vi "Main.vi"() -> ()   [LabVIEW 2019]
uses:
  <vilib>/vision/Image Controls.llb/IMAQ Image.ctl
  <vilib>/vision/NI_Vision_Development_Module.lvlib
panel:
  in  "Save Button":bool
  in  "Clear Button":bool
  in  "Image Path":path=path "Data/(1).jpg" caption="Picture Path"
  in  "Exit":bool
  in  "Start":bool
  out "Results":string
  out "Image":T1(plugin-control)
  # "Application Panel"
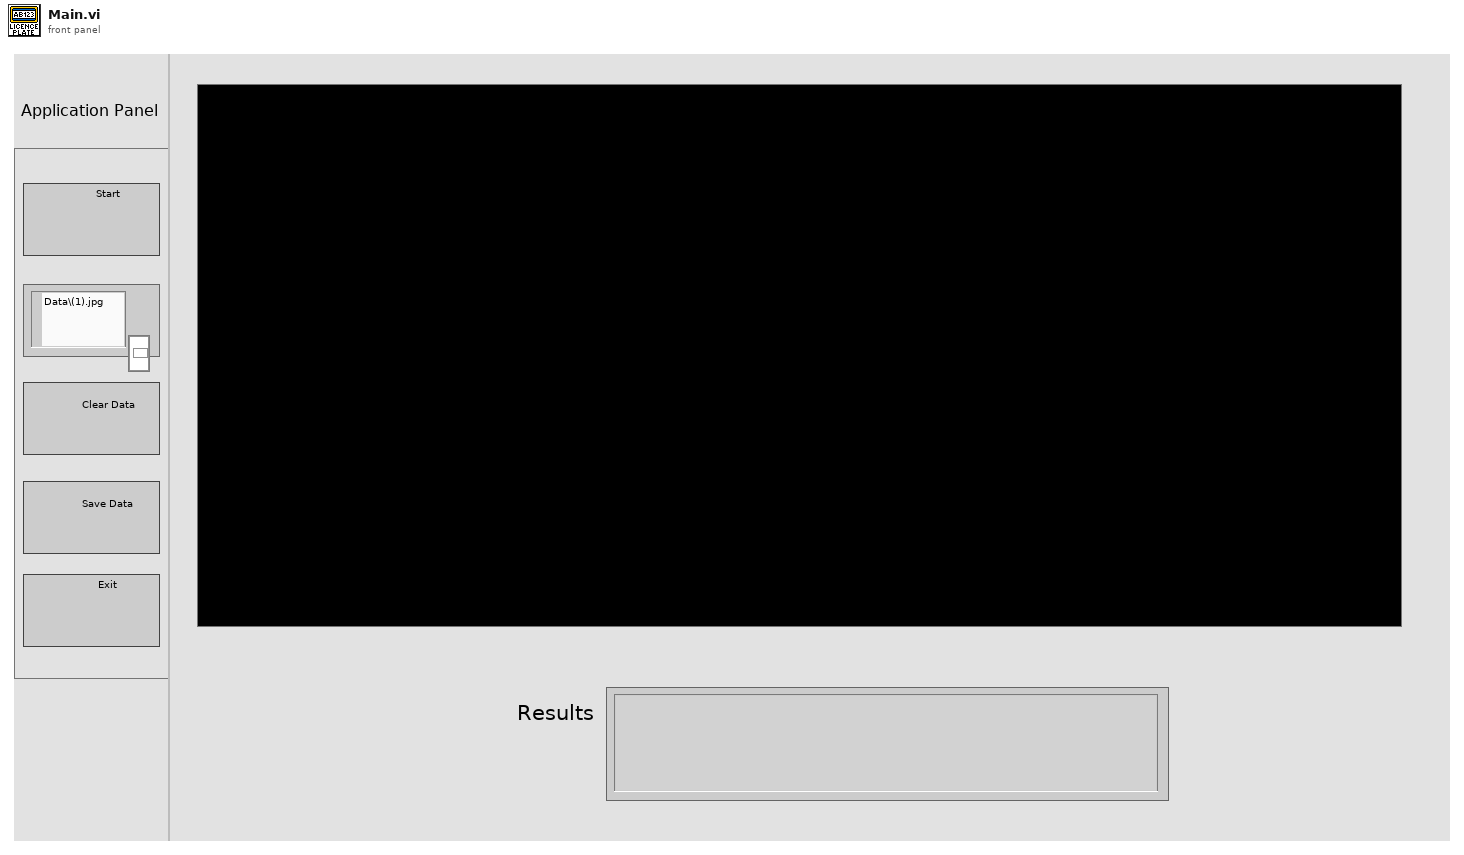
[diagram p1: front panel]
types:
  T1 = typedef "IMAQ Image.ctl" = refnum<image>
  T2 = enum32{"Invalid", "Standard", "Closed", "Hidden", "Minimized", "Maximized"}
  T3 = enum32{"invalid app kind", "Development System", "Run Time System", "Student Edition", "Embedded LabVIEW", "Evaluation", "Custom"}
  T4 = cluster{"Core":cluster{"Current VI Reference":refnum<vi>, "Close Panel on Exit?":bool}, "Your Boolean data":bool, "Results":string, "Image Path":path, "Data":cluster{"Rectangle":i32[]}, "Image":refnum<image>, "Python Path":path}
  T5 = cluster{"Current VI Reference":refnum<vi>, "Close Panel on Exit?":bool}
  T6 = typedef "Image Type" = u32
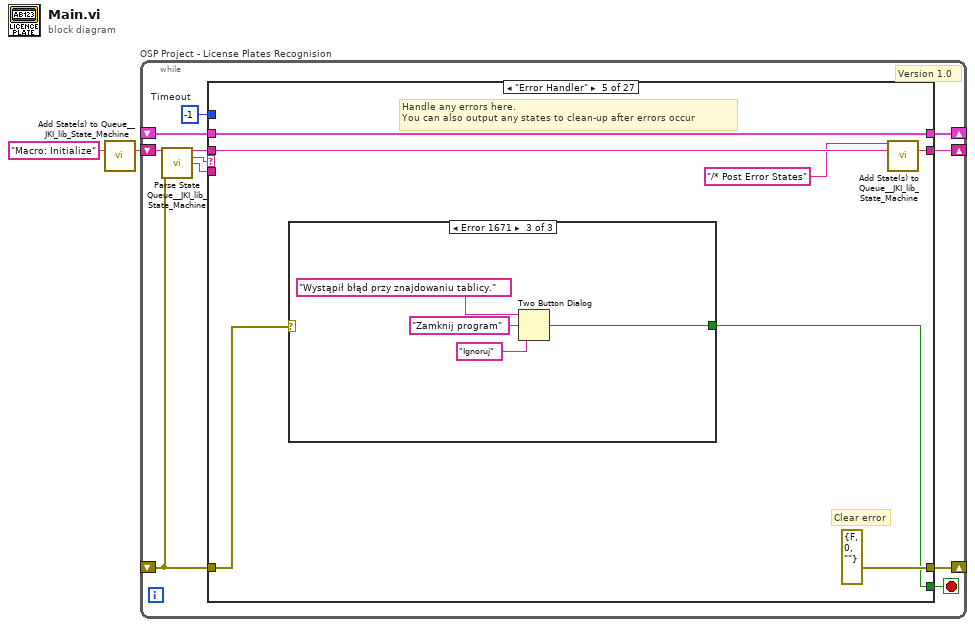
[diagram p0: block diagram]
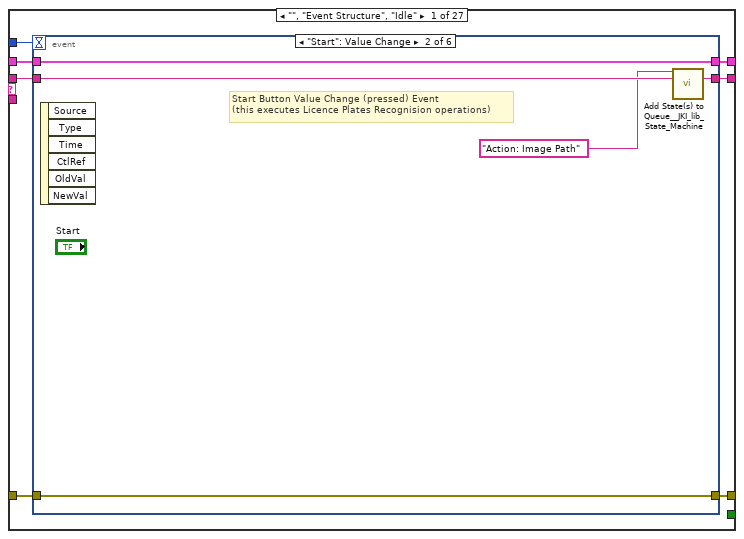
[diagram p2: hidden frame]
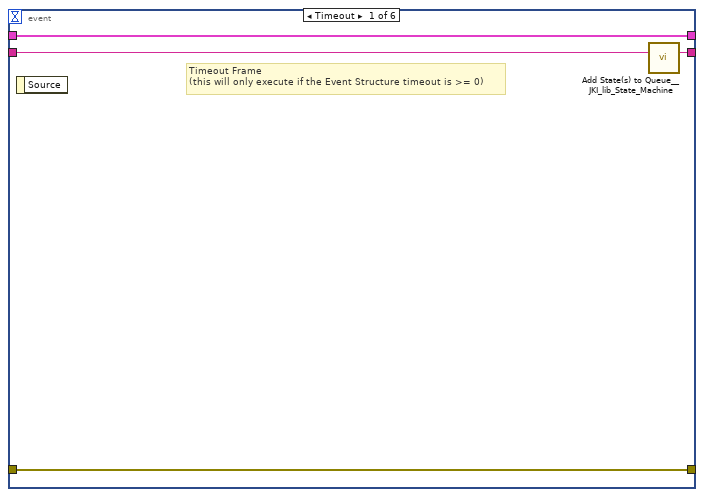
[diagram p3: hidden frame]
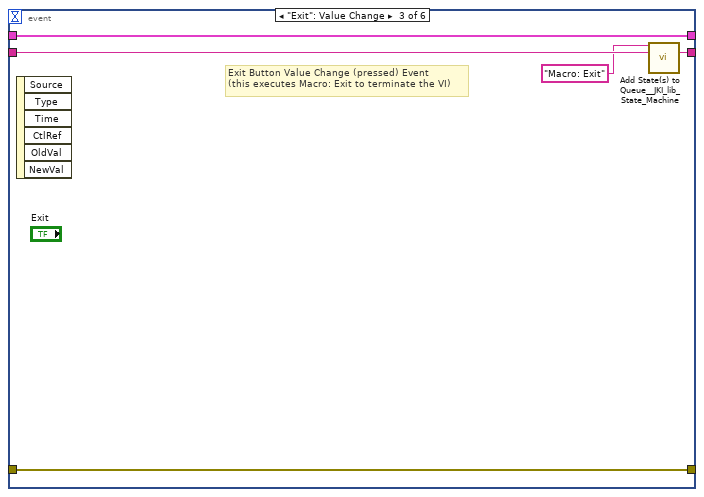
[diagram p4: hidden frame]
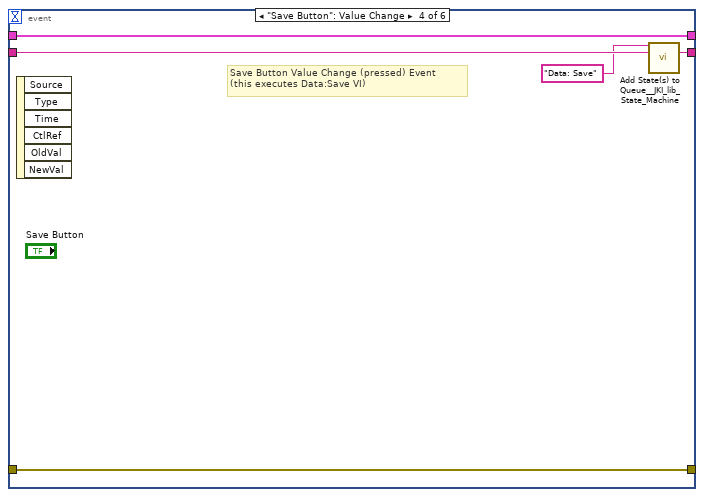
[diagram p5: hidden frame]
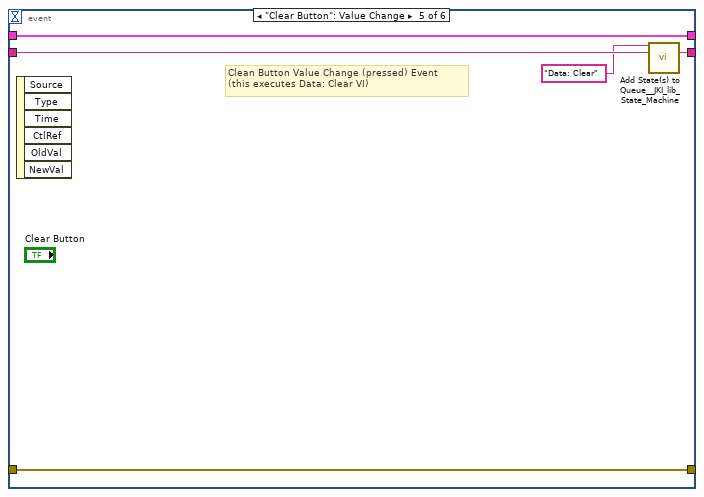
[diagram p6: hidden frame]
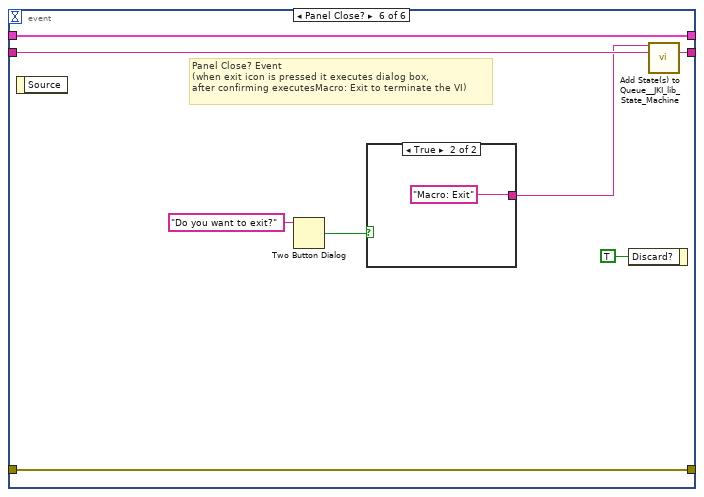
[diagram p7: hidden frame]
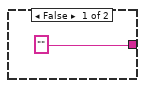
[diagram p8: hidden frame]
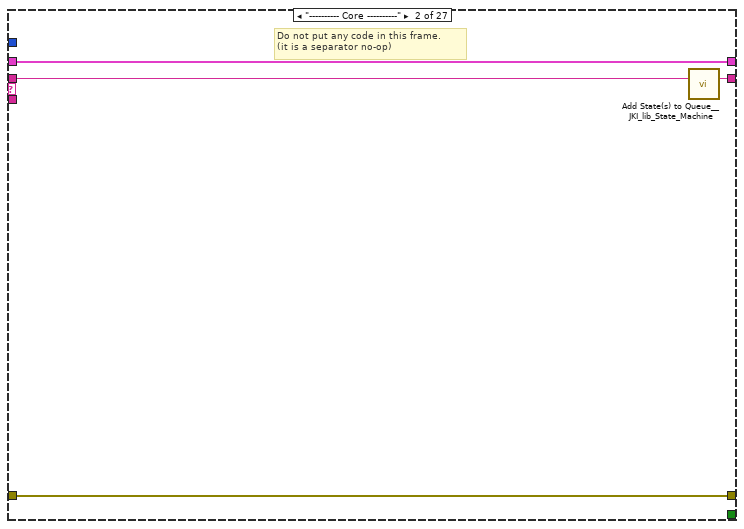
[diagram p9: hidden frame]
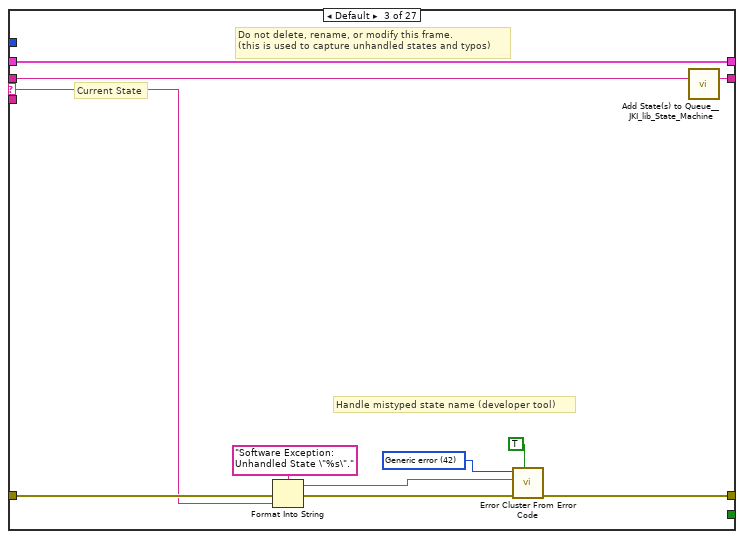
[diagram p10: hidden frame]
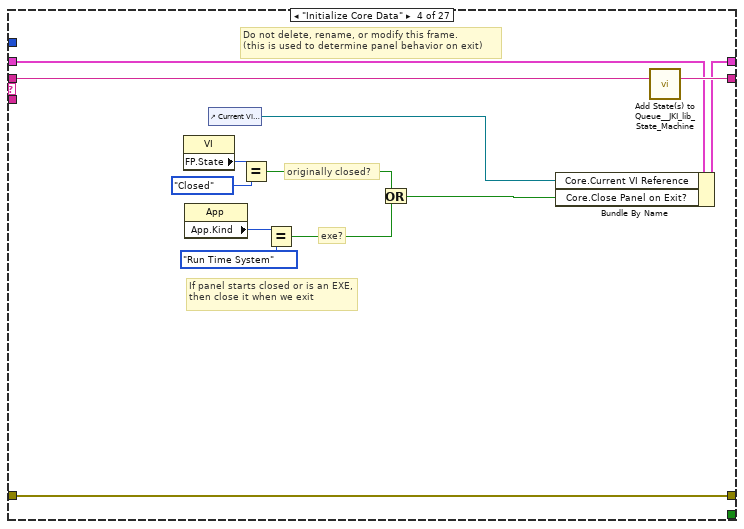
[diagram p11: hidden frame]
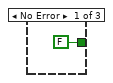
[diagram p12: hidden frame]
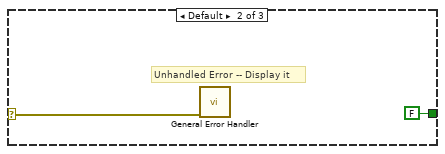
[diagram p13: hidden frame]
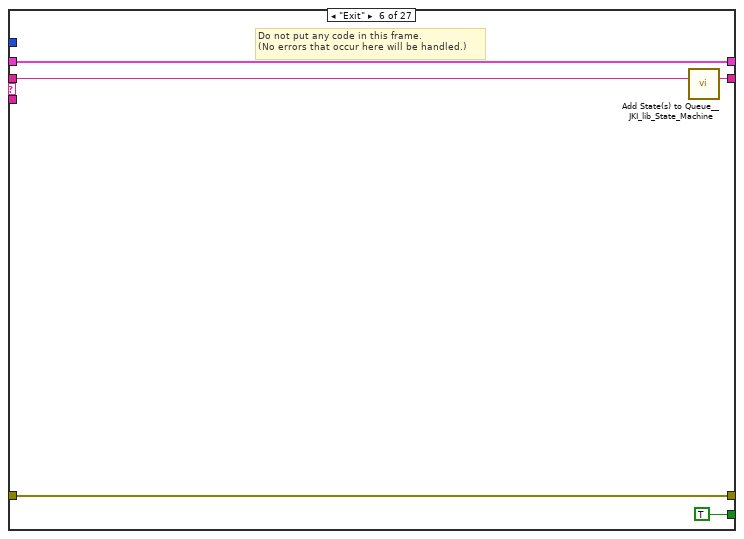
[diagram p14: hidden frame]
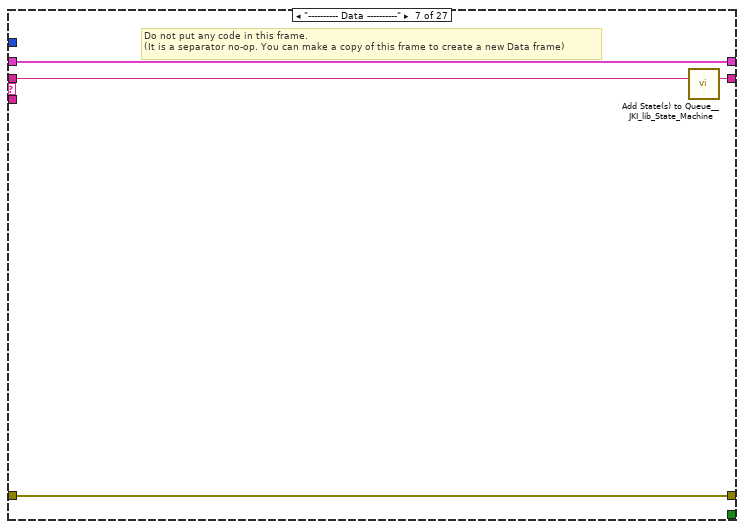
[diagram p15: hidden frame]
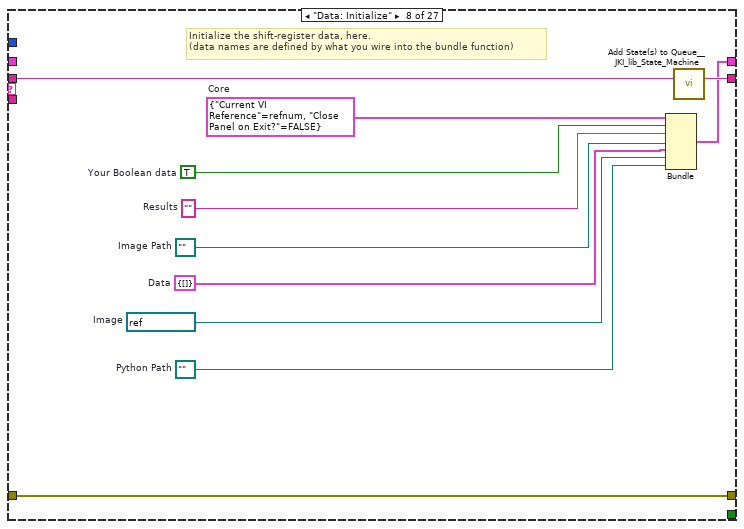
[diagram p16: hidden frame]
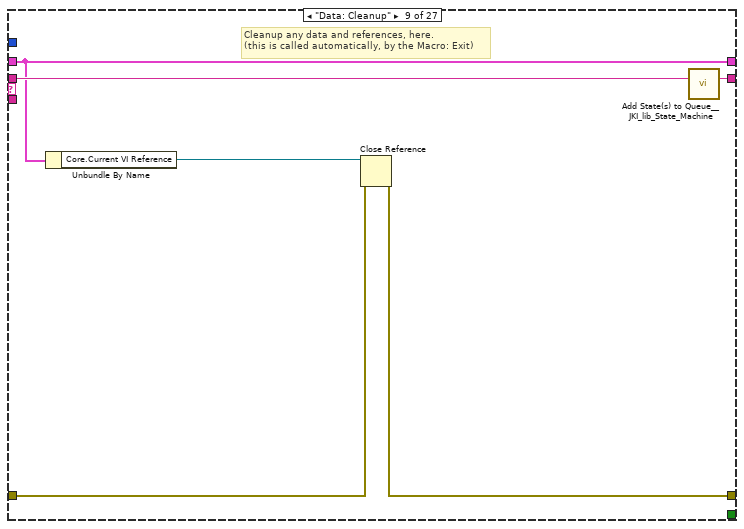
[diagram p17: hidden frame]
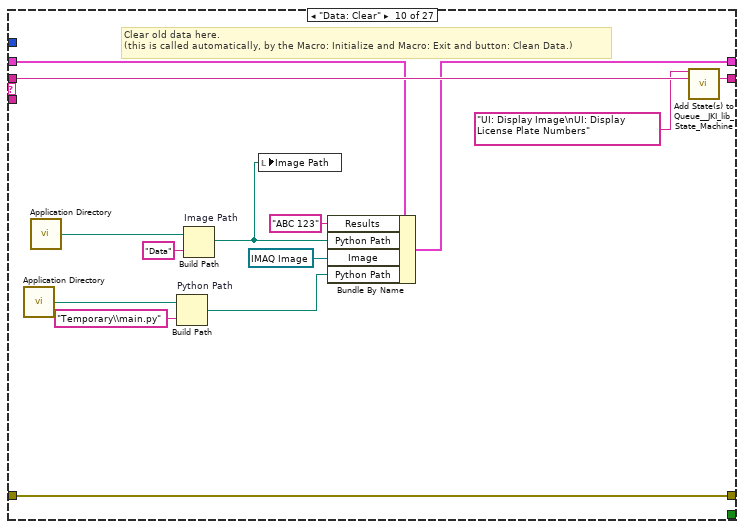
[diagram p18: hidden frame]
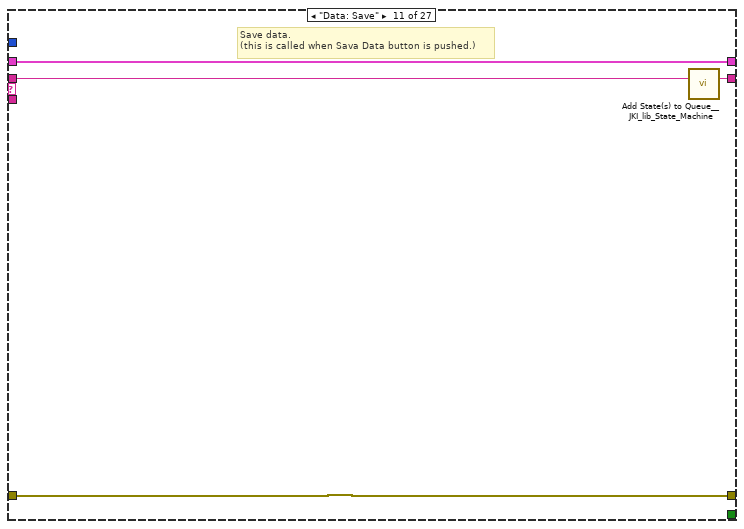
[diagram p19: hidden frame]
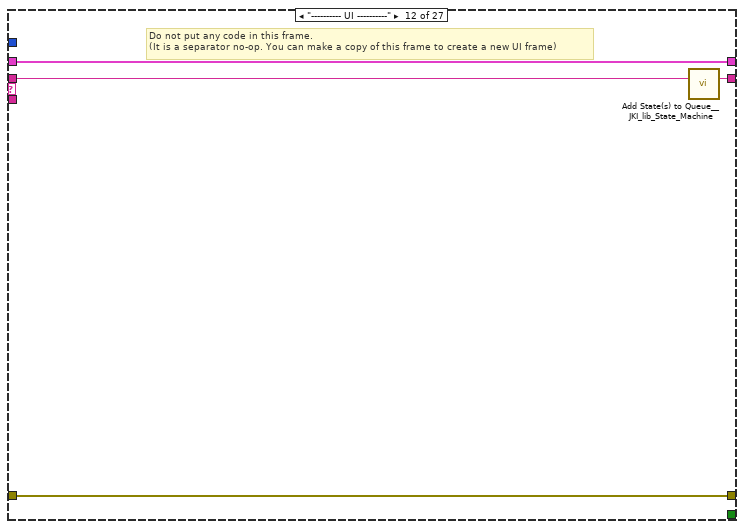
[diagram p20: hidden frame]
diagram:
  n1 = call <vilib>:"Add State(s) to Queue__JKI_lib_State_Machine.vi"("State(s) in (\"\")"="Macro: Initialize") -> ("States Out"=w2:string)  [unwired: 14 in]
  n2 = while "OSP Project - License Plates Recognision" {
    shift-right: [w6] -> _
    shift-left: _ -> [w5]
    shift-right: [w9] -> _
    shift-left: _ -> [w3]
    shift-right: [w8] -> _
    shift-left: w2 -> [w10]
    stop <- w7 stop-if-true
    w4 = -1  # Timeout
    # "Version 1.0"
    n3 = call <vilib>:"Parse State Queue__JKI_lib_State_Machine.vi"("State Queue"=w10, "Error In (no error)"=w3) -> ("Remaining States"=w12:string, "Current State"=w13:string, "Arguments"=w11:string)  [unwired: 11 in]
    n4 = case shown="\"Error Handler\"" w13 {
      selector: w13 -> [_ _ w59 _ _ _ _ _ _ _ _ _ _ _ _ _ _ _ _ _ _ _ _ _ _ _ _]
      tunnel: w12 -> [w20 w58 w63 w82 w89 w101 w105 w116 w122 w136 w140 w144 w148 w154 w165 w235 w240 w244 w249 w259 w263 w273 w300 w309 w318 w329 w338]
      tunnel: w11 -> [_ _ _ _ _ _ _ _ _ _ _ _ _ w149 w159 _ _ _ _ _ _ _ _ _ _ _ _]
      tunnel: w5 -> [w18 w55 w61 w75 w86 w99 w102 _ w117 w132 w138 w141 w146 w152 w161 w232 w237 w241 w246 w256 w260 w269 w288 w303 w313 w321 w332]
      tunnel: [w17 w56 w65 w79 errorcluster {"status"=FALSE, "code"=0, "source"=""} ("error out") w98 w103 w113 w118 w134 w137 w142 w145 w150 w162 w233 w238 w242 w247 w257 w261 w271 w283 w307 w316 w327 w335] -> w9
      tunnel: w3 -> [w16 w56 w64 w79 w84 w98 w103 w113 w119 w134 w137 w142 w145 w151 w163 w233 w238 w242 w247 w257 w261 w271 w286 w307 w316 w327 w334]
      tunnel: [w19 w57 w62 w81 w88 w100 w104 w115 w121 w135 w139 w143 w147 w153 w164 w234 w239 w243 w248 w258 w262 w272 w299 w308 w317 w328 w337] -> w8
      tunnel: [_ _ _ _ w83 TRUE _ _ _ _ _ _ _ _ _ _ _ _ _ _ _ _ _ _ _ _ _] -> w7
      tunnel: [w15 w55 w61 w80 w86 w99 w102 w114 w117 w133 w138 w141 w146 w152 w161 w232 w237 w241 w246 w256 w260 w270 w289 w304 w314 w322 w333] -> w6
      tunnel: w4 -> [w14 _ _ _ _ _ _ _ _ _ _ _ _ _ _ _ _ _ _ _ _ _ _ _ _ _ _]
      frame "", "Event Structure", "Idle" {
        n5 = event shown="[1] \"Start\": Value Change" {
          selector: _ -> [_ _ _ _ _ _]
          dyn-events: _ -> [_ _ _ _ _ _]
          timeout: w14 -> [_ _ _ _ _ _]
          tunnel: w20 -> [w24 w29 w34 w39 w44 w52]
          tunnel: [w23 w28 w33 w38 w43 w51] -> w19
          tunnel: w18 -> [w21 w26 w31 w36 w41 w49]
          tunnel: [w22 w27 w32 w37 w42 w50] -> w17
          tunnel: w16 -> [w22 w27 w32 w37 w42 w50]
          tunnel: [w21 w26 w31 w36 w41 w49] -> w15
          event Timeout {
            # "Timeout Frame\n(this will only execute if the Event Structure timeout is >= 0)"
            n6 = event-data() -> ()  [unwired: 1 in, 1 out]
            n7 = call <vilib>:"Add State(s) to Queue__JKI_lib_State_Machine.vi"("State(s) in (\"\")"=w24) -> ("States Out"=w23:string)  [unwired: 14 in]
          }
          event "Start": Value Change {
            # "Start Button Value Change (pressed) Event\n(this executes Licence Plates Recognision operations)"
            n8 = event-data() -> ()  [unwired: 1 in, 6 out]
            n9 = call <vilib>:"Add State(s) to Queue__JKI_lib_State_Machine.vi"("State(s) in Front (\"\")"="Action: Image Path", "State(s) in (\"\")"=w29) -> ("States Out"=w28:string)  [unwired: 13 in]
          }
          event "Exit": Value Change {
            # "Exit Button Value Change (pressed) Event\n(this executes Macro: Exit to terminate the VI)"
            n10 = event-data() -> ()  [unwired: 1 in, 6 out]
            n11 = call <vilib>:"Add State(s) to Queue__JKI_lib_State_Machine.vi"("State(s) in Front (\"\")"="Macro: Exit", "State(s) in (\"\")"=w34) -> ("States Out"=w33:string)  [unwired: 13 in]
          }
          event "Save Button": Value Change {
            # "Save Button Value Change (pressed) Event\n(this executes Data:Save VI)"
            n12 = event-data() -> ()  [unwired: 1 in, 6 out]
            n13 = call <vilib>:"Add State(s) to Queue__JKI_lib_State_Machine.vi"("State(s) in Front (\"\")"="Data: Save", "State(s) in (\"\")"=w39) -> ("States Out"=w38:string)  [unwired: 13 in]
          }
          event "Clear Button": Value Change {
            # "Clean Button Value Change (pressed) Event\n(this executes Data: Clear VI)"
            n14 = event-data() -> ()  [unwired: 1 in, 6 out]
            n15 = call <vilib>:"Add State(s) to Queue__JKI_lib_State_Machine.vi"("State(s) in Front (\"\")"="Data: Clear", "State(s) in (\"\")"=w44) -> ("States Out"=w43:string)  [unwired: 13 in]
          }
          event Panel Close? {
            # "Panel Close? Event\n(when exit icon is pressed it executes dialog box, \nafter confirming executesMacro: Exit to terminate the VI)"
            n16 = event-data() -> ()  [unwired: 1 in, 1 out]
            n17 = Two Button Dialog(message="Do you want to exit?") -> (T button?=w47:bool)  [unwired: 2 in]
            n18 = case shown="True" w47 {
              tunnel: ["" "Macro: Exit"] -> w45
              frame False {
              }
              frame True {
              }
            }
            n19 = event-data("Discard?"=TRUE) -> ()  [unwired: 1 in, 1 out]
            n20 = call <vilib>:"Add State(s) to Queue__JKI_lib_State_Machine.vi"("State(s) in Front (\"\")"=w45, "State(s) in (\"\")"=w52) -> ("States Out"=w51:string)  [unwired: 13 in]
          }
        }
      }
      frame "---------- Core ----------" {
        # "Do not put any code in this frame.\n(it is a separator no-op)"
        n21 = call <vilib>:"Add State(s) to Queue__JKI_lib_State_Machine.vi"("State(s) in (\"\")"=w58) -> ("States Out"=w57:string)  [unwired: 14 in]
      }
      frame Default {
        w68 = 42 items=["No error", "Argument error", "Memory is full", "Out of zone", "End of file", "File already open", "Generic file I/O error", "File not found", "File permission error", "Disk is full", "Duplicate path", "Too many files open", "System feature not enabled", "Resource file not found", "Cannot add resource", "Resource not found", "Image not found", "Image memory error", "Pen does not exist", "Config type invalid", "Config token not found", "Config parse error", "Config memory error", "Bad external code format", "Bad external code offset", "External code not present", "Null window", "Destroy window error", "Null menu", "Print aborted", "Bad print record", "Print driver error", "Windows error during printing", "Memory error during printing", "Print dialog error", "Generic print error", "Invalid device refnum", "Device not found", "Device parameter error", "Device unit error", "Cannot open device", "Device call aborted", "Generic error", "Cancelled by user", "Object ID too low", "Object ID too high", "Object not in heap", "Unknown heap", "Unknown object (invalid DefProc)", "Unknown object (DefProc not in table)", "Message out of range", "Invalid (null) method", "Unknown message", "Manager call not supported", "Bad address", "Network operation in progress", "Network operation timed out", "Connection is busy", "Network attribute not supported", "Network error", "Address in use", "System out of memory", "Connection aborted", "Connection refused", "Not connected", "Already connected", "Connection closed", "Initialization error (interapplication manager)", "Bad occurrence", "Wait on unbound occurrence handler", "Occurrence queue overflow", "Datalog type conflict", "Unused", "Unrecognized type (interapplication manager)", "Memory corrupt", "Failed to make temporary DLL", "Old CIN version", "Drag socket not found", "Failed to load drop-object", "Failed to register OLE object", "Failed to release OLE object", "Format specifier type mismatch", "Unknown format specifier", "Too few format specifiers", "Too many format specifiers", "Scan failed", "Newer CIN version", "Error converting to variant", "Runtime menu error", "Password tampered", "Variant attribute not found", "Incompatible variant data type", "Event data is not available", "Event Store is not present", "Occurrence is not found", "Event Queue is not created", "Event info is not available", "Refnum passed is NULL", "Error retrieving Class GUID", "Error retrieving CoClass GUID", "Error retrieving TypeLib GUID.", "Bad built application magic bytes.", "Specific driver is different from the specific driver associated with the Logical Name.", "There is no session opened to the class driver.", "Max Error", "MAX - Error with config objects", "MAX - Error loading configuration", "MAX - Group not supported"]
        # "Current State"
        # "Do not delete, rename, or modify this frame.\n(this is used to capture unhandled states and typos)"
        # "Handle mistyped state name (developer tool)"
        n22 = Format Into String(format string="Software Exception: Unhandled State \"%s\"." ("message"), error in=w64, w59) -> (resulting string=w67:string, error out=w66:errorcluster)  [unwired: 1 in]
        n23 = call <vilib>:"Error Cluster From Error Code.vi"("show call chain? (False)"=TRUE, "error in (no error)"=w66, "error message (\"\")"=w67, "error code (0)"=w68) -> ("error out"=w65:errorcluster)  [unwired: 5 in]
        n24 = call <vilib>:"Add State(s) to Queue__JKI_lib_State_Machine.vi"("State(s) in (\"\")"=w63) -> ("States Out"=w62:string)  [unwired: 14 in]
      }
      frame "Initialize Core Data" {
        # "Do not delete, rename, or modify this frame.\n(this is used to determine panel behavior on exit)"
        # "originally closed?"
        # "exe?"
        # "If panel starts closed or is an EXE, then close it when we exit"
        n25 = property class="VI"() -> ("FP.State"=w72:T2)  [unwired: 2 in, 2 out]
        n26 = property class="App"() -> ("App.Kind"=w78:T3)  [unwired: 2 in, 2 out]
        n27 = control-ref of="Current VI Reference"() -> (w73:refnum<vi>)
        n28 = Equal?(x=w72, y=T2."Closed" ("Front Panel Window:State")) -> (x = y?=w70:bool)
        n29 = Equal?(x=w78, y=T3."Run Time System" ("Application:Kind")) -> (x = y?=w76:bool)
        n30 = Or(x=w70, y=w76) -> (x .or. y?=w74:bool)
        n31 = Bundle By Name(cluster=w75, "Core.Current VI Reference"=w73, "Core.Close Panel on Exit?"=w74) -> (w80:T4)
        n32 = call <vilib>:"Add State(s) to Queue__JKI_lib_State_Machine.vi"("State(s) in (\"\")"=w82) -> ("States Out"=w81:string)  [unwired: 14 in]
      }
      frame "Error Handler" {
        # "Handle any errors here.\nYou can also output any states to clean-up after errors occur"
        # "Clear error"
        n33 = case shown="Error 1671" w84 {
          selector: w84 -> [_ w91 _]
          tunnel: [FALSE ("T button?") FALSE ("T button?") w95] -> w83
          frame No Error {
          }
          frame Default {
            # "Unhandled Error -- Display it"
            n34 = call <vilib>:"General Error Handler.vi"("error in (no error)"=w91) -> ()  [unwired: 10 in, 5 out]
          }
          frame Error {
            n35 = Two Button Dialog(message="Wystąpił błąd przy znajdowaniu tablicy.", 1:"Ignoruj" ("F button name (\"Cancel\")"), 2:"Zamknij program" ("T button name (\"OK\")")) -> (T button?=w95:bool)
          }
        }
        n36 = call <vilib>:"Add State(s) to Queue__JKI_lib_State_Machine.vi"("State(s) in Front (\"\")"="/* Post Error States", "State(s) in (\"\")"=w89) -> ("States Out"=w88:string)  [unwired: 13 in]
      }
      frame "Exit" {
        # "Do not put any code in this frame.\n(No errors that occur here will be handled.)"
        n37 = call <vilib>:"Add State(s) to Queue__JKI_lib_State_Machine.vi"("State(s) in (\"\")"=w101) -> ("States Out"=w100:string)  [unwired: 14 in]
      }
      frame "---------- Data ----------" {
        # "Do not put any code in this frame.\n(It is a separator no-op. You can make a copy of this frame to create a new Data frame)"
        n38 = call <vilib>:"Add State(s) to Queue__JKI_lib_State_Machine.vi"("State(s) in (\"\")"=w105) -> ("States Out"=w104:string)  [unwired: 14 in]
      }
      frame "Data: Initialize" {
        w106 = path ""  # Python Path
        w107 = path ""  # Image Path
        w108 = refnum<image> refnum  # Image
        w109 = cluster{"Rectangle":i32[]} {"Rectangle"=[]}  # Data
        w110 = T5 {"Current VI Reference"=refnum, "Close Panel on Exit?"=FALSE}  # Core
        w112 = TRUE  # Your Boolean data
        w111 = ""  # Results
        # "Initialize the shift-register data, here.\n(data names are defined by what you wire into the bundle function)"
        n39 = Bundle("Core"=w110, "Your Boolean data"=w112, "Results"=w111, "Image Path"=w107, "Data"=w109, "Image"=w108, "Python Path"=w106) -> (w114:T4)  [unwired: 1 in]
        n40 = call <vilib>:"Add State(s) to Queue__JKI_lib_State_Machine.vi"("State(s) in (\"\")"=w116) -> ("States Out"=w115:string)  [unwired: 14 in]
      }
      frame "Data: Cleanup" {
        # "Cleanup any data and references, here.\n(this is called automatically, by the Macro: Exit)"
        n41 = Unbundle By Name(w117) -> ("Core.Current VI Reference"=w120:refnum<vi>)
        n42 = Close Reference(reference=w120, error in (no error)=w119) -> (error out=w118:errorcluster)
        n43 = call <vilib>:"Add State(s) to Queue__JKI_lib_State_Machine.vi"("State(s) in (\"\")"=w122) -> ("States Out"=w121:string)  [unwired: 14 in]
      }
      frame "Data: Clear" {
        # "Clear old data here.\n(this is called automatically, by the Macro: Initialize and Macro: Exit and button: Clean Data.)"
        n44 = call <vilib>:"Application Directory.vi"() -> ("Application Directory"=w125:path)
        n45 = call <vilib>:"Application Directory.vi"() -> ("Application Directory"=w128:path)
        n46 = Build Path "Python Path"(base path=w125, name or relative path="Temporary\\main.py") -> (appended path=w123:path)
        n47 = Build Path "Image Path"(base path=w128, name or relative path="Data") -> (appended path=w126:path)
        n48 = local write "Image Path"(w126) -> ()
        n49 = Bundle By Name(cluster=w132, "Results"="ABC 123", "Python Path"=w126, "Image"=T1 refnum, "Python Path"=w123) -> (w133:T4)
        n50 = call <vilib>:"Add State(s) to Queue__JKI_lib_State_Machine.vi"("State(s) in Front (\"\")"="UI: Display Image\nUI: Display License Plate Numbers", "State(s) in (\"\")"=w136) -> ("States Out"=w135:string)  [unwired: 13 in]
      }
      frame "Data: Save" {
        # "Save data.\n(this is called when Sava Data button is pushed.)"
        n51 = call <vilib>:"Add State(s) to Queue__JKI_lib_State_Machine.vi"("State(s) in (\"\")"=w140) -> ("States Out"=w139:string)  [unwired: 14 in]
      }
      frame "---------- UI ----------" {
        # "Do not put any code in this frame.\n(It is a separator no-op. You can make a copy of this frame to create a new UI frame)"
        n52 = call <vilib>:"Add State(s) to Queue__JKI_lib_State_Machine.vi"("State(s) in (\"\")"=w144) -> ("States Out"=w143:string)  [unwired: 14 in]
      }
      frame "UI: Initialize" {
        # "Initialize the User Interface, here.\n(this is called automatically, by the Macro: Init)"
        n53 = call <vilib>:"Add State(s) to Queue__JKI_lib_State_Machine.vi"("State(s) in (\"\")"=w148) -> ("States Out"=w147:string)  [unwired: 14 in]
      }
      frame "UI: Cursor Set" {
        # "Argument"
        # "Set and Unset Cursor Busy.\n(Usage: \"UI: Cursor Set >> Busy|Idle\")"
        n54 = case shown="\"Idle\", Default" w149 {
          tunnel: w151 -> [w156 w158]
          tunnel: [w155 w157] -> w150
          frame "Idle", Default {
            n55 = call <vilib>:"Unset Busy.vi"("error in (no error)"=w156) -> ("error out"=w155:errorcluster)  [unwired: 10 in]
          }
          frame "Busy" {
            n56 = call <vilib>:"Set Busy.vi"("error in (no error)"=w158) -> ("error out"=w157:errorcluster)  [unwired: 9 in, 1 out]
          }
        }
        n57 = call <vilib>:"Add State(s) to Queue__JKI_lib_State_Machine.vi"("State(s) in (\"\")"=w154) -> ("States Out"=w153:string)  [unwired: 14 in]
      }
      frame "UI: Front Panel State" {
        # "Argument"
        # "Set Front Panel Open or Closed\n(Usage: \"UI: Front Panel State >> Open|Close\")"
        n58 = Unbundle By Name(w161) -> ("Core.Current VI Reference"=w160:refnum<vi>)
        n59 = case shown="\"Minimize\", \"Minimized\"" w159 {
          tunnel: w163 -> [w171 w186 w197 w210 w223]
          tunnel: [w173 w187 w199 w212 w225] -> w162
          tunnel: w160 -> [w172 w184 w198 w211 w224]
          frame "Open", "Standard", Default {
            w166 = T2."Standard" ("State")
            n60 = property class="VI"(reference=w172, error in=w171) -> (reference out=w169:refnum<vi>, error out=w170:errorcluster, "FP.State"=w168:T2)
            n61 = Not Equal?(x=w168, y=w166) -> (x != y?=w167:bool)
            n62 = case shown="True" w167 {
              tunnel: [w177 w179] -> w173
              tunnel: w170 -> [w176 w179]
              tunnel: w169 -> [w175 _]
              tunnel: w166 -> [w174 _]
              frame True {
                n63 = invoke class="VI" method="FP.Open"(reference=w175, error in=w176, "Activate"=TRUE, "State"=w174) -> (error out=w177:errorcluster)  [unwired: 1 in, 4 out]
              }
              frame False {
              }
            }
          }
          frame "Close", "Closed" {
            n64 = property class="VI"(reference=w184, error in=w186) -> (reference out=w183:refnum<vi>, error out=w185:errorcluster, "FP.State"=w181:T2)
            n65 = Not Equal?(x=w181, y=T2."Closed" ("Front Panel Window:State")) -> (x != y?=w180:bool)
            n66 = case shown="True" w180 {
              tunnel: [w188 w191] -> w187
              tunnel: w185 -> [w188 w190]
              tunnel: w183 -> [_ w189]
              frame False {
              }
              frame True {
                n67 = invoke class="VI" method="FP.Close"(reference=w189, error in=w190) -> (error out=w191:errorcluster)  [unwired: 1 in, 2 out]
              }
            }
          }
          frame "Hidden", "Hide" {
            w192 = T2."Hidden" ("State")
            n68 = property class="VI"(reference=w198, error in=w197) -> (reference out=w195:refnum<vi>, error out=w196:errorcluster, "FP.State"=w194:T2)
            n69 = Not Equal?(x=w194, y=w192) -> (x != y?=w193:bool)
            n70 = case shown="True" w193 {
              tunnel: [w203 w204] -> w199
              tunnel: w196 -> [w202 w204]
              tunnel: w195 -> [w201 _]
              tunnel: w192 -> [w200 _]
              frame True {
                n71 = invoke class="VI" method="FP.Open"(reference=w201, error in=w202, "State"=w200) -> (error out=w203:errorcluster)  [unwired: 2 in, 4 out]
              }
              frame False {
              }
            }
          }
          frame "Minimize", "Minimized" {
            w205 = T2."Minimized" ("State")
            n72 = property class="VI"(reference=w211, error in=w210) -> (reference out=w208:refnum<vi>, error out=w209:errorcluster, "FP.State"=w207:T2)
            n73 = Not Equal?(x=w207, y=w205) -> (x != y?=w206:bool)
            n74 = case shown="True" w206 {
              tunnel: [w216 w217] -> w212
              tunnel: w209 -> [w215 w217]
              tunnel: w208 -> [w214 _]
              tunnel: w205 -> [w213 _]
              frame True {
                n75 = invoke class="VI" method="FP.Open"(reference=w214, error in=w215, "State"=w213) -> (error out=w216:errorcluster)  [unwired: 2 in, 4 out]
              }
              frame False {
              }
            }
          }
          frame "Maximize", "Maximized" {
            w218 = T2."Maximized" ("State")
            n76 = property class="VI"(reference=w224, error in=w223) -> (reference out=w221:refnum<vi>, error out=w222:errorcluster, "FP.State"=w220:T2)
            n77 = Not Equal?(x=w220, y=w218) -> (x != y?=w219:bool)
            n78 = case shown="True" w219 {
              tunnel: [w229 w230] -> w225
              tunnel: w222 -> [w228 w230]
              tunnel: w221 -> [w227 _]
              tunnel: w218 -> [w226 _]
              frame True {
                n79 = invoke class="VI" method="FP.Open"(reference=w227, error in=w228, "State"=w226) -> (error out=w229:errorcluster)  [unwired: 2 in, 4 out]
              }
              frame False {
              }
            }
          }
        }
        n80 = call <vilib>:"Add State(s) to Queue__JKI_lib_State_Machine.vi"("State(s) in (\"\")"=w165) -> ("States Out"=w164:string)  [unwired: 14 in]
      }
      frame "UI: Display Image" {
        # "Display Image\n(In this frame Image is displayed on UI.)"
        n81 = Unbundle By Name(w232) -> ("Image"=→"Image":refnum<image>)
        n82 = call <vilib>:"Add State(s) to Queue__JKI_lib_State_Machine.vi"("State(s) in (\"\")"=w235) -> ("States Out"=w234:string)  [unwired: 14 in]
      }
      frame "UI: Display License Plate Numbers" {
        # "Display License Plate Numbers\n(In this frame Resoults are displayed on UI.)"
        n83 = Unbundle By Name(w237) -> ("Results"=→"Results":string)
        n84 = call <vilib>:"Add State(s) to Queue__JKI_lib_State_Machine.vi"("State(s) in (\"\")"=w240) -> ("States Out"=w239:string)  [unwired: 14 in]
      }
      frame "---------- Macro ----------" {
        # "Do not put any code in this frame.\n(It is a separator no-op. You can make a copy of this frame to create a new Macro frame)"
        n85 = call <vilib>:"Add State(s) to Queue__JKI_lib_State_Machine.vi"("State(s) in (\"\")"=w244) -> ("States Out"=w243:string)  [unwired: 14 in]
      }
      frame "Macro: Initialize" {
        w245 = "Data: Initialize\nInitialize Core Data\nData: Clear\nUI: Initialize\nUI: Front Panel State >> Open"  # Data: Initialize Initialize Core Data Data: Clear UI: Initialize UI: Front Panel State >> Open
        # "Initialization Macro\n(This is called once, when the VI starts)"
        n86 = call <vilib>:"Add State(s) to Queue__JKI_lib_State_Machine.vi"("State(s) in Front (\"\")"=w245, "State(s) in (\"\")"=w249) -> ("States Out"=w248:string)  [unwired: 13 in]
      }
      frame "Macro: Exit" {
        # "Exit Macro\n(This is called once, when the VI exits)"
        n87 = Unbundle By Name(w256) -> ("Core.Close Panel on Exit?"=w255:bool)
        n88 = Select(t="UI: Front Panel State >> Close", s=w255, f="") -> (s? t:f=w252:string)
        n89 = call <vilib>:"Add State(s) to Queue__JKI_lib_State_Machine.vi"("State(s) in (\"\")"=w252, "State(s) at Back (\"\")"="Data: Cleanup\nData: Clear\nExit") -> ("States Out"=w250:string)  [unwired: 13 in]
        n90 = call <vilib>:"Add State(s) to Queue__JKI_lib_State_Machine.vi"("State(s) in Front (\"\")"=w250, "State(s) in (\"\")"=w259) -> ("States Out"=w258:string)  [unwired: 13 in]
      }
      frame "---------- Action ----------" {
        # "Template Separator\n(You can make a copy of, or modify, this frame)"
        n91 = call <vilib>:"Add State(s) to Queue__JKI_lib_State_Machine.vi"("State(s) in (\"\")"=w263) -> ("States Out"=w262:string)  [unwired: 14 in]
      }
      frame "Action: Image Path" {
        w268 = path ""  # Empty Path Constant
        # "Image Path.\n(Checking if Image Path is correct.)"
        n92 = Equal?(x="Image Path", y=w268) -> (x = y?=w267:bool)
        n93 = case shown="True" w267 {
          tunnel: "Image Path" -> [w276 _]
          tunnel: [w277 TRUE] -> w264
          frame False {
            w278 = "jpg" ("search string/char (-)")
            n94 = Path To String(path=w276) -> (string=w279:string)
            n95 = Search/Split String(string=w279, search string/char (-)=w278) -> (match + rest of string=w280:string)  [unwired: 1 in, 2 out]
            n96 = Equal?(x=w280, y=w278) -> (x = y?=w277:bool)
          }
          frame True {
            n97 = One Button Dialog(message="Image path is EMPTY!\nPlease select image path.") -> ()  [unwired: 1 in, 1 out]
          }
        }
        n98 = Bundle By Name(cluster=w269, "Image Path"="Image Path") -> (w270:T4)
        n99 = case shown="False" w264 {
          tunnel: [_ "Action: Python Code"] -> w265
          frame False {
            n100 = One Button Dialog(message="Image path is NOT CORRECT!\nPlease select JPG image.") -> ()  [unwired: 1 in, 1 out]
          }
          frame True {
          }
        }
        n101 = call <vilib>:"Add State(s) to Queue__JKI_lib_State_Machine.vi"("State(s) in Front (\"\")"=w265, "State(s) in (\"\")"=w273) -> ("States Out"=w272:string)  [unwired: 13 in]
      }
      frame "Action: Python Code" {
        w295 = "find_plate"  # function name
        w298 = "3.6"  # Python version
        # "Python Code.\n(In this frame we are using Python Node to identify coordinates of license plate.)"
        n102 = Unbundle By Name(w288) -> ("Image Path"=w291:path)
        n103 = Unbundle By Name(w288) -> ("Data.Rectangle"=w293:i32[])
        n104 = Unbundle By Name(w288) -> ("Python Path"=w292:path)
        n105 = Open Python Session(python version=w298, 3:w286) -> (session out=w297:refnum<k35>, error out=w285:errorcluster)  [unwired: 1 in]
        n106 = Path To String(path=w291) -> (string=w294:string)
        n107 = node(w297, w292, w295, w285, w293, w294) -> (w296:refnum<k35>, w284:errorcluster, w290:i32[])  [unwired: 1 in, 2 out]
        n108 = Close Python Session(session in=w296, error in=w284) -> (11:w283:errorcluster)
        n109 = Bundle By Name(cluster=w288, "Data.Rectangle"=w290) -> (w289:T4)
        n110 = call <vilib>:"Add State(s) to Queue__JKI_lib_State_Machine.vi"("State(s) in Front (\"\")"="Action: IMAQ Create" ("State(s) in Front (\"\")"), "State(s) in (\"\")"=w300) -> ("States Out"=w299:string)  [unwired: 13 in]
      }
      frame "Action: IMAQ Create" {
        w305 = T6 4 items=["Grayscale (U8)", "Grayscale (I16)", "Grayscale (SGL)", "Complex (CSG)", "RGB (U32)", "HSL (U32)", "RGB (U64)", "Grayscale (U16)"] ("Image Type")
        w306 = "untitled"  # Image Name
        # "IMAQ Create.\n(In this frame it is created a temorary memory location for an image.)"
        n111 = call "IMAQ Create"("Image Name"=w306, "Image Type"=w305) -> ("New Image"=w302:T1)  [unwired: 3 in, 1 out]
        n112 = Bundle By Name(cluster=w303, "Image"=w302) -> (w304:T4)
        n113 = call <vilib>:"Add State(s) to Queue__JKI_lib_State_Machine.vi"("State(s) in Front (\"\")"="Action: IMAQ Read FIle" ("State(s) in Front (\"\")"), "State(s) in (\"\")"=w309) -> ("States Out"=w308:string)  [unwired: 13 in]
      }
      frame "Action: IMAQ Read FIle" {
        # "IMAQ Read File.\n(In this frame image file is being read.)"
        n114 = Unbundle By Name(w313) -> ("Image"=w312:refnum<image>)
        n115 = Unbundle By Name(w313) -> ("Image Path"=w315:path)
        n116 = call "IMAQ ReadFile 2.vi"("File Path"=w315, "Image"=w312) -> ("Image Out"=w310:T1)  [unwired: 5 in, 4 out]
        n117 = Bundle By Name(cluster=w313, "Image"=w310) -> (w314:T4)
        n118 = call <vilib>:"Add State(s) to Queue__JKI_lib_State_Machine.vi"("State(s) in Front (\"\")"="Action: IMAQ Extract" ("State(s) in Front (\"\")"), "State(s) in (\"\")"=w318) -> ("States Out"=w317:string)  [unwired: 13 in]
      }
      frame "Action: IMAQ Extract" {
        w319 = 1  # Y Step Size
        w325 = 1  # X Step Size
        # "IMAQ Extract.\n(In this frame part of image is extracted with adjustment of the horizontal and vertical resolution.)"
        n119 = Unbundle By Name(w321) -> ("Data.Rectangle"=w324:i32[])
        n120 = Unbundle By Name(w321) -> ("Image"=w326:refnum<image>)
        n121 = call "IMAQ Extract 2"("Y Step Size"=w319, "Optional Rectangle"=w324, "X Step Size"=w325, "Image Src"=w326) -> ("Image Dst Out"=w323:T1)  [unwired: 6 in, 1 out]
        n122 = Bundle By Name(cluster=w321, "Image"=w323) -> (w322:T4)
        n123 = call <vilib>:"Add State(s) to Queue__JKI_lib_State_Machine.vi"("State(s) in Front (\"\")"="UI: Display Image\nAction: IMAQ OCR", "State(s) in (\"\")"=w329) -> ("States Out"=w328:string)  [unwired: 13 in]
      }
      frame "Action: IMAQ OCR" {
        # "IMAQ OCR.\n(In this frame the optical character recognition is being used.)"
        n124 = Unbundle By Name(w332) -> ("Image"=w336:refnum<image>)
        n125 = call "IMAQ OCR.vi"("Image In"=w336, "error in"=w334) -> ("String (OCR/OCV 2)"=w331:string, "error out"=w335:errorcluster)  [unwired: 24 in]
        n126 = Bundle By Name(cluster=w332, "Results"=w331) -> (w333:T4)
        n127 = call <vilib>:"Add State(s) to Queue__JKI_lib_State_Machine.vi"("State(s) in Front (\"\")"="UI: Display License Plate Numbers" ("State(s) in Front (\"\")"), "State(s) in (\"\")"=w338) -> ("States Out"=w337:string)  [unwired: 13 in]
      }
    }
  }
